vi "Find Delimited String.vi"(0 "String":string, 5 "Delimiter Regular Expression ([\\r\\n])":string="[\\r\\n]", 7 "Start Offset (0)":u32, 9 "End Offset (0)":u32) -> (4 "Substring":string, 8 "Location":T1)   [LabVIEW 2016, in "Code String.lvclass"]
doc: "Using the given <b>Delimiter Regular Expression</b>, returns the <b>Substring<b> in <b>String</b> bounded by <b>Start</b> and <b>End</b> that is between the delimiter(s). Looks for the first delimiter before <b>Start Offset</b> and after <b>End Offset</b>. Also returns the <b>Location</b> in <b>String</b> where <b>Substring</b> was found.\n--------------------\nCopyright (c) 2019 Analog Devices, Inc. All rights reserved.\n\nRedistribution and use in source and binary forms, with or without modification,\nare permitted provided that the following conditions are met:\n - Redistributions of source code must retain the above copyright notice, this\n list of conditions and the following disclaimer.\n - Redistributions in binary form must reproduce the above copyright notice,\n this list of conditions and the following disclaimer in the documentation\n and/or other materials provided with the distribution.\n - Modified versions of the software must be conspicuously marked as such.\n - This software is licensed solely and exclusively for use with\n processors/products manufactured by or for Analog Devices, Inc.\n - This software may not be combined or merged with other code in any manner\n that would cause the software to become subject to terms and conditions\n which differ from those listed here.\n - Neither the name of Analog Devices, Inc. nor the names of its contributors\n may be used to endorse or promote products derived from this software\n without specific prior written permission.\n - The use of this software may or may not infringe the patent rights of one or\n more patent holders. This license does not release you from the requirement\n that you obtain separate licenses from these patent holders to use this\n software.\n\nTHIS SOFTWARE IS PROVIDED BY ANALOG DEVICES, INC. AND CONTRIBUTORS \"AS IS\" AND\nANY EXPRESS OR IMPLIED WARRANTIES, INCLUDING, BUT NOT LIMITED TO,\nNON-INFRINGEMENT, TITLE, MERCHANTABILITY AND FITNESS FOR A PARTICULAR PURPOSE\nARE DISCLAIMED. IN NO EVENT SHALL ANALOG DEVICES, INC. OR CONTRIBUTORS BE LIABLE\nFOR ANY DIRECT, INDIRECT, INCIDENTAL, SPECIAL, EXEMPLARY, PUNITIVE OR\nCONSEQUENTIAL DAMAGES (INCLUDING, BUT NOT LIMITED TO, DAMAGES ARISING OUT OF\nCLAIMS OF INTELLECTUAL PROPERTY RIGHTS INFRINGEMENT; PROCUREMENT OF SUBSTITUTE\nGOODS OR SERVICES; LOSS OF USE, DATA, OR PROFITS; OR BUSINESS INTERRUPTION)\nHOWEVER CAUSED AND ON ANY THEORY OF LIABILITY, WHETHER IN CONTRACT, STRICT\nLIABILITY, OR TORT (INCLUDING NEGLIGENCE OR OTHERWISE) ARISING IN ANY WAY OUT OF\nTHE USE OF THIS SOFTWARE, EVEN IF ADVISED OF THE POSSIBILITY OF SUCH DAMAGE.\n\n2019-01-10-7CBSD SLA"
uses:
  Code String.lvclass
  <vilib>/Utility/miscctls.llb/LVSelectionTypeDef.ctl
panel:
  # "Copyright (c) 2019 Analog Devices, Inc.  All rights reserved.\n\nRedistribution and use in source and binary forms, with or without modification,\nare permitted provided that the following conditions are met:\n  - Redistributions of source code must retain the above copyright notice, this\n    list of conditions and the following disclaimer.\n  - Redistributions in binary form must reproduce the above copyright notice,\n    this list of conditions and the following disclaimer in the documentation\n    and/or other materials provided with the distribution.\n  - Modified versions of the software must be conspicuously marked as such.\n  - This software is licensed solely and exclusively for use with\n    processors/products manufactured by or for Analog Devices, Inc.\n  - This software may not be combined or merged with other code in any manner\n    that would cause the software to become subject to terms and conditions\n    which differ from those listed here.\n  - Neither the name of Analog Devices, Inc. nor the names of its contributors\n    may be used to endorse or promote products derived from this software\n    without specific prior written permission.\n  - The use of this software may or may not infringe the patent rights of one or\n    more patent holders.  This license does not release you from the requirement\n    that you obtain separate licenses from these patent holders to use this\n    software.\n\nTHIS SOFTWARE IS PROVIDED BY ANALOG DEVICES, INC. AND CONTRIBUTORS \"AS IS\" AND\nANY EXPRESS OR IMPLIED WARRANTIES, INCLUDING, BUT NOT LIMITED TO,\nNON-INFRINGEMENT, TITLE, MERCHANTABILITY AND FITNESS FOR A PARTICULAR PURPOSE\nARE DISCLAIMED. IN NO EVENT SHALL ANALOG DEVICES, INC. OR CONTRIBUTORS BE LIABLE\nFOR ANY DIRECT, INDIRECT, INCIDENTAL, SPECIAL, EXEMPLARY, PUNITIVE OR\nCONSEQUENTIAL DAMAGES (INCLUDING, BUT NOT LIMITED TO, DAMAGES ARISING OUT OF\nCLAIMS OF INTELLECTUAL PROPERTY RIGHTS INFRINGEMENT; PROCUREMENT OF SUBSTITUTE\nGOODS OR SERVICES; LOSS OF USE, DATA, OR PROFITS; OR BUSINESS INTERRUPTION)\nHOWEVER CAUSED AND ON ANY THEORY OF LIABILITY, WHETHER IN CONTRACT, STRICT\nLIABILITY, OR TORT (INCLUDING NEGLIGENCE OR OTHERWISE) ARISING IN ANY WAY OUT OF\nTHE USE OF THIS SOFTWARE, EVEN IF ADVISED OF THE POSSIBILITY OF SUCH DAMAGE.\n\n2019-01-10-7CBSD SLA"
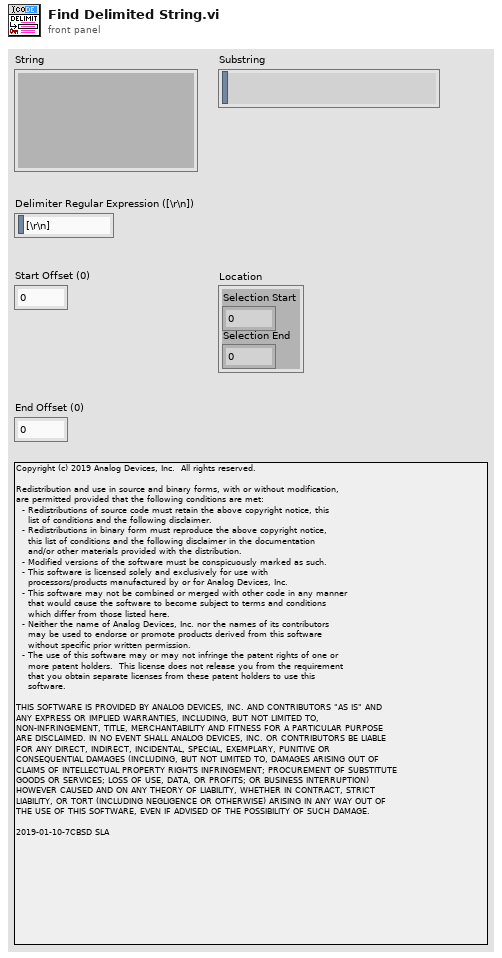
[diagram p1: front panel]
types:
  T1 = typedef "LVSelectionTypeDef.ctl" = cluster{"Selection Start":u32, "Selection End":u32}
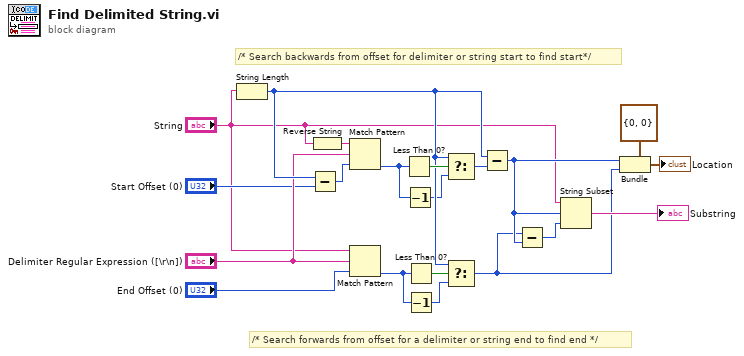
[diagram p0: block diagram]
diagram:
  # "/* Search forwards from offset for a delimiter or string end to find end */"
  # "/* Search backwards from offset for delimiter or string start to find start*/"
  n1 = String Length(string="String") -> (length=w13:i32)
  n2 = Subtract(x=w13, y="Start Offset (0)") -> (x-y=w19:u32)
  n3 = Reverse String(1:"String") -> (0:w20:string)
  n4 = Match Pattern(string=w20, regular expression="Delimiter Regular Expression ([\\r\\n])", offset (0)=w19) -> (offset past match=w12:i32)  [unwired: 3 out]
  n5 = Match Pattern(string="String", regular expression="Delimiter Regular Expression ([\\r\\n])", offset (0)="End Offset (0)") -> (offset past match=w14:i32)  [unwired: 3 out]
  n6 = Less Than 0?(x=w12) -> (x < 0?=w17:bool)
  n7 = Decrement(x=w12) -> (x-1=w9:i32)
  n8 = Less Than 0?(x=w14) -> (x < 0?=w15:bool)
  n9 = Decrement(x=w14) -> (x-1=w10:i32)
  n10 = Select(t=w13, s=w17, f=w9) -> (s? t:f=w16:i32)
  n11 = Select(t=w13, s=w15, f=w10) -> (s? t:f=w4:i32)
  n12 = Subtract(x=w13, y=w16) -> (x-y=w5:i32)
  n13 = Subtract(x=w4, y=w5) -> (x-y=w18:i32)
  n14 = String Subset(string="String", offset (0)=w5, length (rest)=w18) -> (substring=→"Substring":string)
  n15 = Bundle(cluster=T1 {"Selection Start"=0, "Selection End"=0} ("Text.Selection"), "Selection Start"=w5, "Selection End"=w4) -> (→"Location":T1)
